vi "流量计UI.vi"() -> ()   [LabVIEW 2016, in "流量计集成.lvlib"]
uses:
  <vilib>/Plasmionique/MB Master/MB_Master_Serial/MB_Master_Serial.lvclass
  C:/Program Files (x86)/National Instruments/LabVIEW 2016/vi.lib/Plasmionique/MB Master/MB_Master/MB_Master.lvclass
  <vilib>/Analysis/baseanly.llb/Mean (DBL).vi
  <vilib>/Utility/config.llb/NI_LVConfig.lvlib
  <vilib>/Analysis/NI_AALBase.lvlib
panel:
  in  "流量计启用 4":bool
  in  "数量 4":u16
  out "流量计类型 4":T1=enum."博意达流量计"
  out "平均水位":dbl
  out "总累积流量":dbl
  out "平均流速":dbl
  out "总流量":dbl
  in  "选项卡控件":T2(tab)
  out "数组":T3[](array[typedef])
  out "数组 2":T4[](array[typedef]) {"累积流量单位" items=["L", "M3", "T", "USG"]; "瞬时流量单位" items=["L/S", "L/M", "L/H", "M3/S", "M3/M", "M3/H", "T/S", "T/M", "T/H", "GPS", "GPM", "GPH"]}
  out "数组 3":T7[](array[typedef])
  out "数组 4":T3[](array[typedef])
  out "MB_Serial session":refnum<class "MB_Master_Serial.lvclass">
  in  "斯坦道功率测流":bool
  in  "流量计启用 3":bool
  in  "数量 3":u16
  out "流量计类型 3":T1=enum."斯坦道功率测流"
  in  "流量计启用 2":bool
  in  "数量 2":u16
  out "流量计类型 2":T1=enum."MGG/KL QC"
  in  "数量":u16
  out "流量计类型":T1
  in  "流量计启用":bool
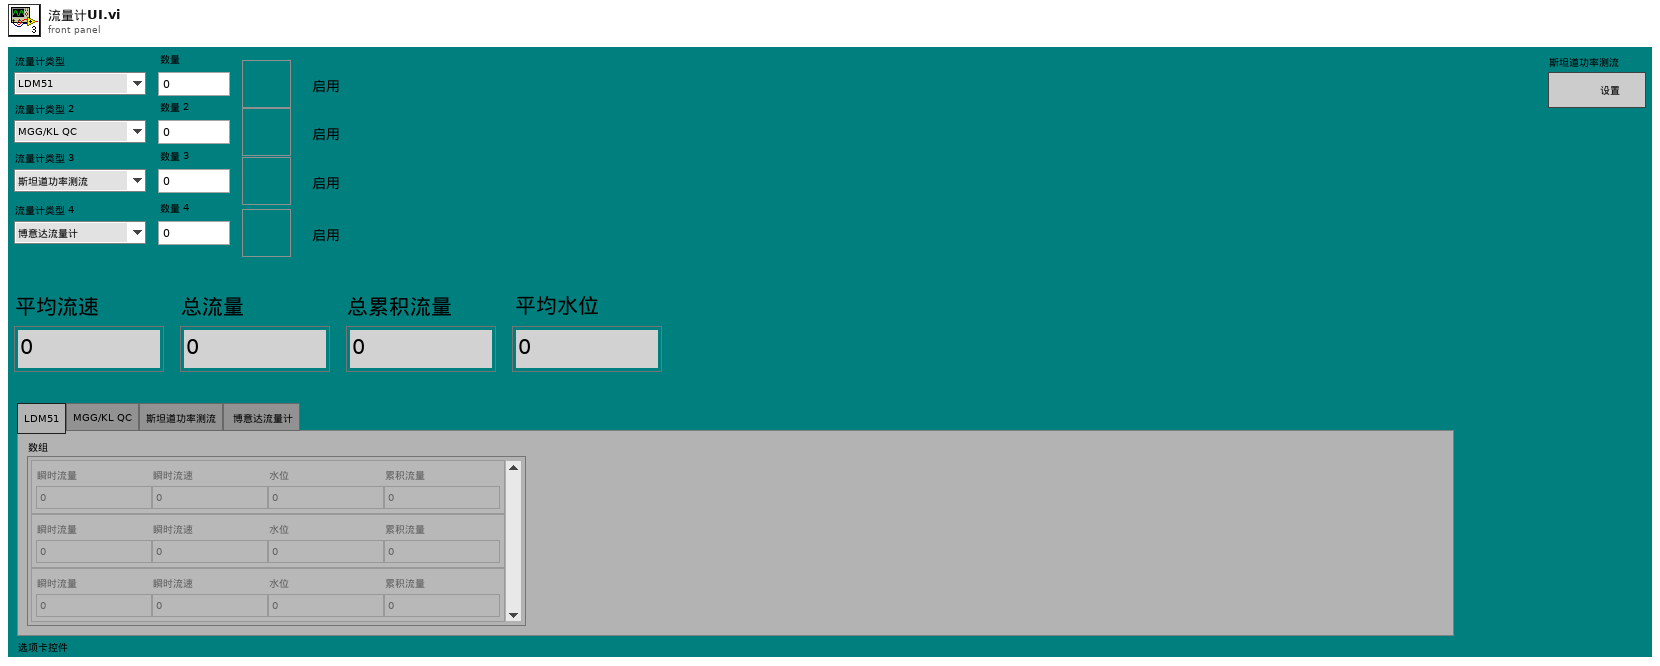
[diagram p1: front panel]
types:
  T1 = typedef "流量计集成.lvlib/流量计类型.ctl" = enum16{"LDM51", "MGG/KL QC", "斯坦道功率测流", "博意达流量计"}
  T2 = enum32{"LDM51", "MGG/KL QC", "斯坦道功率测流", " 博意达流量计"}
  T3 = typedef "流量计集成.lvlib/LDM51明渠流量计.lvlib/读取值.ctl" = cluster{"瞬时流量":sgl, "瞬时流速":sgl, "水位":sgl, "累积流量":sgl}
  T4 = typedef "流量计集成.lvlib/MGG-KL-QC流量计.lvlib/读取值.ctl" = cluster{"瞬时流量":sgl, "瞬时流速":sgl, "流量百分比":sgl, "流体电导比":sgl, "正向累积数值":sgl, "反向累积数值":sgl, "瞬时流量单位":T5, "累积流量单位":T6, "上限报警":u16, "下限报警":u16, "空管报警":u16, "系统报警":u16}
  T5 = typedef "流量计集成.lvlib/MGG-KL-QC流量计.lvlib/瞬时流量单位.ctl" = u16
  T6 = typedef "流量计集成.lvlib/MGG-KL-QC流量计.lvlib/累积流量单位.ctl" = u16
  T7 = typedef "流量计集成.lvlib/斯坦道功率测流.lvlib/状态值.ctl" = cluster{"1号瞬时流量":dbl, "2号瞬时流量":dbl, "3号瞬时流量":dbl, "4号瞬时流量":dbl, "5号瞬时流量":dbl, "6号瞬时流量":dbl, "1号累积流量":dbl, "2号累积流量":dbl, "3号累积流量":dbl, "4号累积流量":dbl, "5号累积流量":dbl, "6号累积流量":dbl, "总瞬时流量":dbl, "总累积流量":dbl}
  T8 = cluster{"时间标识":timestamp, "测量模式":string, "数据类型":string, "监测值":sgl, "单位":string, "数据标识":string, "因子编码":string}
  T9 = typedef "LVDateTimeRec.ctl" = cluster{"秒数的小数部分":dbl, "秒":i32, "分":i32, "时":i32, "日":i32, "月":i32, "年":i32, "天数（周）":i32, "天数（年）":i32, "DST":i32}
  T10 = typedef "流量计集成.lvlib/博意达流量计.lvlib/读取值.ctl" = cluster{"瞬时流量":sgl, "瞬时流速":sgl, "水位":sgl, "累积流量":sgl}
  T11 = typedef "NI_LVConfig.lvlib/Config Data RefNum.ctl" = refnum<k1>
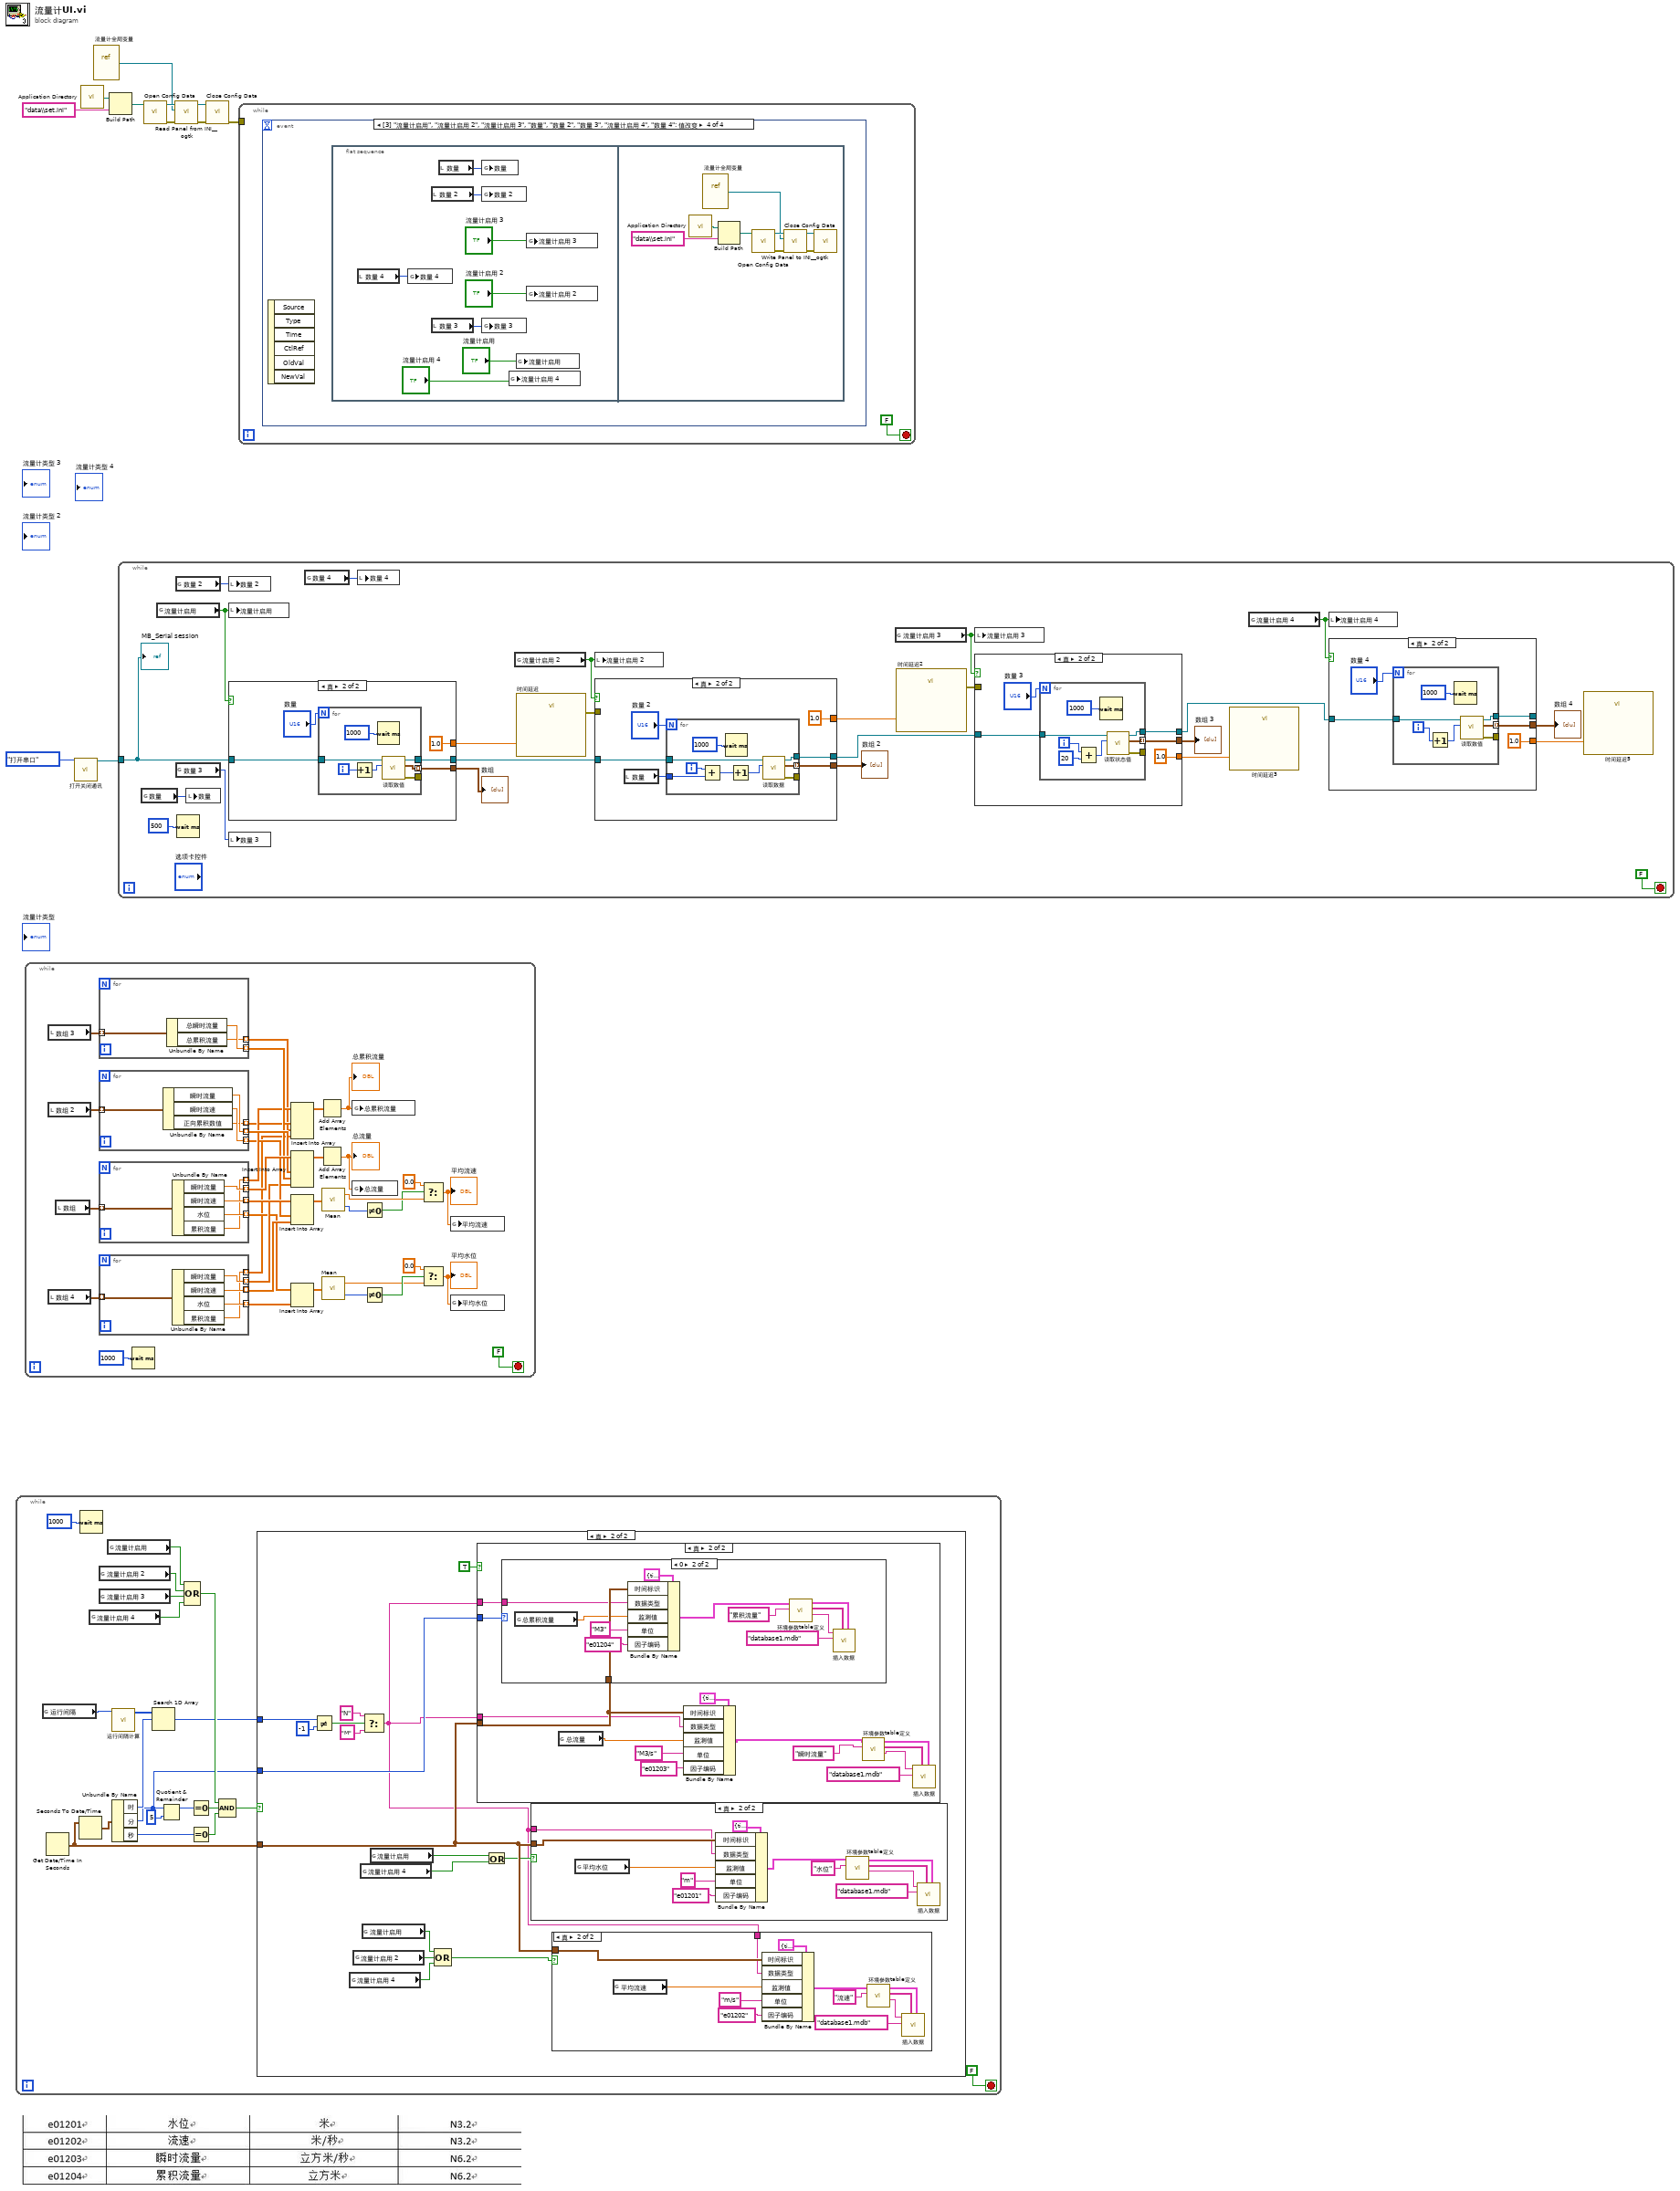
[diagram p0: block diagram]
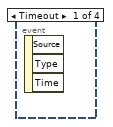
[diagram p7: hidden frame]
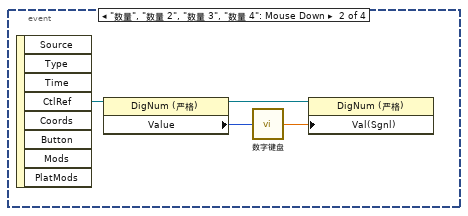
[diagram p8: hidden frame]
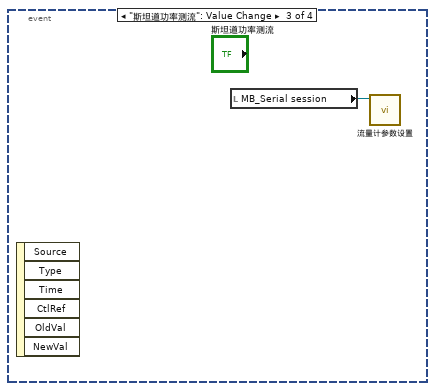
[diagram p9: hidden frame]
diagram:
  n1 = while {
    stop <- FALSE stop-if-true
    n2 = global read "流量计全局变量.vi" "运行间隔"() -> (w13:i16)
    n3 = Get Date/Time In Seconds() -> (seconds since 1Jan1904=w30:timestamp)
    n4 = Seconds To Date/Time(time stamp (now)=w30) -> (date time rec=w29:T9)  [unwired: 1 in]
    n5 = Wait (ms)(milliseconds to wait=u32 1000 ("等待时间（毫秒）")) -> ()  [unwired: 1 out]
    n6 = global read "流量计全局变量.vi" "流量计启用 4"() -> (w12:bool)
    n7 = global read "流量计全局变量.vi" "流量计启用 2"() -> (w20:bool)
    n8 = global read "流量计全局变量.vi" "流量计启用 3"() -> (w19:bool)
    n9 = global read "流量计全局变量.vi" "流量计启用"() -> (w21:bool)
    n10 = call "运行间隔计算.vi"("运行周期"=w13) -> ("数组"=w16:i32[])  [unwired: 10 in]
    n11 = Unbundle By Name(w29) -> ("时"=w17:i32, "分"=w14:i32, "秒"=w27:i32)
    n12 = Search 1D Array(1D array=w16, element=w17) -> (index of element=w15:i32)  [unwired: 1 in]
    n13 = Quotient & Remainder(x=w14, y=5) -> (x-y*floor(x/y)=w26:i32)  [unwired: 1 out]
    n14 = Compound Arithmetic op=OR ("复合运算")(w21, w20, w19, w12) -> (w18:bool)
    n15 = Equal To 0?(x=w26) -> (x = 0?=w25:bool)
    n16 = Equal To 0?(x=w27) -> (x = 0?=w24:bool)
    n17 = Compound Arithmetic op=AND ("复合运算")(w18, w25, w24) -> (w23:bool)
    n18 = case shown="真" w23 {
      tunnel: w30 -> [_ w47]
      tunnel: w15 -> [_ w38]
      tunnel: w14 -> [_ w37]
      frame False {
      }
      frame True {
        n19 = Not Equal?(x=w38, y=-1) -> (x != y?=w41:bool)
        n20 = global read "流量计全局变量.vi" "流量计启用 4"() -> (w35:bool)
        n21 = global read "流量计全局变量.vi" "流量计启用 2"() -> (w43:bool)
        n22 = global read "流量计全局变量.vi" "流量计启用 4"() -> (w33:bool)
        n23 = global read "流量计全局变量.vi" "流量计启用"() -> (w44:bool)
        n24 = Select(t="N" ("单位"), s=w41, f="M" ("单位")) -> (s? t:f=w36:string)
        n25 = global read "流量计全局变量.vi" "流量计启用"() -> (w46:bool)
        n26 = Compound Arithmetic op=OR ("复合运算")(w44, w43, w35) -> (w32:bool)
        n27 = case shown="真" TRUE {
          tunnel: w47 -> [_ w68]
          tunnel: w36 -> [_ w72]
          tunnel: w37 -> [_ w71]
          tunnel: w36 -> [_ w66]
          frame False {
          }
          frame True {
            n28 = case shown="0" w71 {
              tunnel: w68 -> [_ w84]
              tunnel: w72 -> [_ w81]
              frame Default {
              }
              frame 0 {
                n29 = global read "流量计全局变量.vi" "总累积流量"() -> (w82:dbl)
                n30 = Bundle By Name(cluster=T8 {"时间标识"=timestamp(0 s since 1904-01-01), "测量模式"="水样测试", "数据类型"="N", "监测值"=0.0, "单位"="mg/L", "数据标识"="N", "因子编码"=""} ("data"), "时间标识"=w84, "数据类型"=w81, "监测值"=w82, "单位"="M3", "因子编码"="e01204") -> (w78:T8)
                n31 = call "环境参数table定义.vi"("table 输入"="累积流量", "data"=w78) -> ("table 输出"=w74:string, "columns"=w75:string[], "data输出"=w76:T8)  [unwired: 7 in]
                n32 = call "插入数据.vi"("data"=w76, "columns"=w75, "database"="database1.mdb" ("table 输入"), "table"=w74) -> ()  [unwired: 7 in, 1 out]
              }
            }
            n33 = global read "流量计全局变量.vi" "总流量"() -> (w67:dbl)
            n34 = Bundle By Name(cluster=T8 {"时间标识"=timestamp(0 s since 1904-01-01), "测量模式"="水样测试", "数据类型"="N", "监测值"=0.0, "单位"="mg/L", "数据标识"="N", "因子编码"=""} ("data"), "时间标识"=w68, "数据类型"=w66, "监测值"=w67, "单位"="M3/s", "因子编码"="e01203") -> (w64:T8)
            n35 = call "环境参数table定义.vi"("table 输入"="瞬时流量", "data"=w64) -> ("table 输出"=w60:string, "columns"=w61:string[], "data输出"=w62:T8)  [unwired: 7 in]
            n36 = call "插入数据.vi"("data"=w62, "columns"=w61, "database"="database1.mdb" ("table 输入"), "table"=w60) -> ()  [unwired: 7 in, 1 out]
          }
        }
        n37 = Or(x=w46, y=w33) -> (x .or. y?=w45:bool)
        n38 = case shown="真" w45 {
          tunnel: w47 -> [_ w55]
          tunnel: w36 -> [_ w54]
          frame False {
          }
          frame True {
            n39 = global read "流量计全局变量.vi" "平均水位"() -> (w53:dbl)
            n40 = Bundle By Name(cluster=T8 {"时间标识"=timestamp(0 s since 1904-01-01), "测量模式"="水样测试", "数据类型"="N", "监测值"=0.0, "单位"="mg/L", "数据标识"="N", "因子编码"=""} ("data"), "时间标识"=w55, "数据类型"=w54, "监测值"=w53, "单位"="m", "因子编码"="e01201") -> (w49:T8)
            n41 = call "环境参数table定义.vi"("table 输入"="水位", "data"=w49) -> ("table 输出"=w50:string, "columns"=w51:string[], "data输出"=w52:T8)  [unwired: 7 in]
            n42 = call "插入数据.vi"("data"=w52, "columns"=w51, "database"="database1.mdb" ("table 输入"), "table"=w50) -> ()  [unwired: 7 in, 1 out]
          }
        }
        n43 = case shown="真" w32 {
          tunnel: w47 -> [_ w92]
          tunnel: w36 -> [_ w91]
          frame False {
          }
          frame True {
            n44 = global read "流量计全局变量.vi" "平均流速"() -> (w93:dbl)
            n45 = Bundle By Name(cluster=T8 {"时间标识"=timestamp(0 s since 1904-01-01), "测量模式"="水样测试", "数据类型"="N", "监测值"=0.0, "单位"="mg/L", "数据标识"="N", "因子编码"=""} ("data"), "时间标识"=w92, "数据类型"=w91, "监测值"=w93, "单位"="m/s", "因子编码"="e01202") -> (w89:T8)
            n46 = call "环境参数table定义.vi"("table 输入"="流速", "data"=w89) -> ("table 输出"=w86:string, "columns"=w87:string[], "data输出"=w88:T8)  [unwired: 7 in]
            n47 = call "插入数据.vi"("data"=w88, "columns"=w87, "database"="database1.mdb" ("table 输入"), "table"=w86) -> ()  [unwired: 7 in, 1 out]
          }
        }
      }
    }
  }
  n48 = while {
    stop <- FALSE stop-if-true
    n49 = local read "数组 3"() -> (w128:T7[])
    n50 = local read "数组 2"() -> (w129:T4[])
    n51 = local read "数组 4"() -> (w104:T3[])
    n52 = local read "数组"() -> (w132:T3[])
    n53 = for {
      tunnel: w128 -> [w140] mode=indexing
      tunnel: [w139] -> w125 mode=indexing
      tunnel: [w138] -> w122 mode=indexing
      n54 = Unbundle By Name(w140) -> ("总瞬时流量"=w139:dbl, "总累积流量"=w138:dbl)
    }
    n55 = for {
      tunnel: w129 -> [w144] mode=indexing
      tunnel: [w143] -> w126 mode=indexing
      tunnel: [w142] -> w118 mode=indexing
      tunnel: [w141] -> w123 mode=indexing
      n56 = Unbundle By Name(w144) -> ("瞬时流量"=w143:sgl, "瞬时流速"=w142:sgl, "正向累积数值"=w141:sgl)
    }
    n57 = for {
      tunnel: w132 -> [w149] mode=indexing
      tunnel: [w148] -> w127 mode=indexing
      tunnel: [w147] -> w119 mode=indexing
      tunnel: [w146] -> w101 mode=indexing
      tunnel: [w145] -> w124 mode=indexing
      n58 = Unbundle By Name(w149) -> ("瞬时流量"=w148:sgl, "瞬时流速"=w147:sgl, "水位"=w146:sgl, "累积流量"=w145:sgl)
    }
    n59 = for {
      tunnel: w104 -> [w137] mode=indexing
      tunnel: [w136] -> w102 mode=indexing
      tunnel: [w135] -> w103 mode=indexing
      tunnel: [w134] -> w99 mode=indexing
      tunnel: [w133] -> w98 mode=indexing
      n60 = Unbundle By Name(w137) -> ("瞬时流量"=w136:sgl, "瞬时流速"=w135:sgl, "水位"=w134:sgl, "累积流量"=w133:sgl)
    }
    n61 = Wait (ms)(milliseconds to wait=u32 1000 ("等待时间（毫秒）")) -> ()  [unwired: 1 out]
    n62 = Insert Into Array(array=w124, new element #1=w123, new element #2=w122, new element #3=w98) -> (w120:sgl[])  [unwired: 1 in]
    n63 = Insert Into Array(array=w127, new element #1=w126, new element #2=w125, new element #3=w102) -> (w121:sgl[])  [unwired: 1 in]
    n64 = Insert Into Array(array=w119, new element #1=w118, new element #2=w103) -> (w113:sgl[])  [unwired: 1 in]
    n65 = Insert Into Array(array=w101, new element=w99) -> (w100:sgl[])  [unwired: 1 in]
    n66 = Add Array Elements(numeric array=w120) -> (sum=w106:sgl)
    "总累积流量" <- w106
    n67 = Add Array Elements(numeric array=w121) -> (sum=w108:sgl)
    "总流量" <- w108
    n68 = call-poly <vilib>:"Mean.vi"("X"=w113) -> ("mean"=w117:dbl, "error"=w114:i32)
    n69 = call-poly <vilib>:"Mean.vi"("X"=w100) -> ("mean"=w109:dbl, "error"=w112:i32)
    n70 = global write "流量计全局变量.vi" "总累积流量"(w106) -> ()
    n71 = global write "流量计全局变量.vi" "总流量"(w108) -> ()
    n72 = Not Equal To 0?(x=w114) -> (x != 0?=w115:bool)
    n73 = Not Equal To 0?(x=w112) -> (x != 0?=w111:bool)
    n74 = Select(t=0.0, s=w115, f=w117) -> (s? t:f=w107:dbl)
    "平均流速" <- w107
    n75 = Select(t=0.0, s=w111, f=w109) -> (s? t:f=w105:dbl)
    "平均水位" <- w105
    n76 = global write "流量计全局变量.vi" "平均流速"(w107) -> ()
    n77 = global write "流量计全局变量.vi" "平均水位"(w105) -> ()
  }
  n78 = call "打开关闭通讯.vi"("功能输入"=enum16{"打开串口", "关闭串口"}."打开串口") -> ("MB_Serial session"=w1:refnum<class "MB_Master_Serial.lvclass">)  [unwired: 9 in, 1 out]
  n79 = call <vilib>:"Application Directory.vi"() -> ("Application Directory"=w9:path)
  n80 = vi-ref "流量计全局变量.vi"() -> (w3:refnum<vi>)
  n81 = Build Path(base path=w9, name or relative path="data\\set.ini" ("名称或相对路径")) -> (appended path=w10:path)
  n82 = while {
    tunnel: w1 -> [w163]
    stop <- FALSE stop-if-true
    n83 = global read "流量计全局变量.vi" "数量"() -> (w162:u16)
    n84 = global read "流量计全局变量.vi" "流量计启用"() -> (w171:bool)
    n85 = global read "流量计全局变量.vi" "数量 2"() -> (w161:u16)
    n86 = global read "流量计全局变量.vi" "数量 3"() -> (w160:u16)
    n87 = Wait (ms)(milliseconds to wait=u32 500 ("等待时间（毫秒）")) -> ()  [unwired: 1 out]
    n88 = local write "数量"(w162) -> ()
    n89 = local write "数量 2"(w161) -> ()
    n90 = local write "流量计启用"(w171) -> ()
    n91 = case shown="真" w171 {
      tunnel: w163 -> [w217 w222]
      tunnel: [w217 w220] -> w170
      tunnel: [_ w219] -> w168
      tunnel: [_ 1.0 ("Delay Time (s)")] -> w159
      frame False {
      }
      frame True {
        n92 = for {
          N: "数量" -> [_]
          tunnel: w222 -> [w229]
          tunnel: [w228] -> _
          tunnel: [w225] -> w220
          tunnel: [w224] -> w219 mode=indexing
          i -> [w227]
          n93 = Increment(x=w227) -> (x+1=w226:i32)
          n94 = Wait (ms)(milliseconds to wait=u32 1000 ("等待时间（毫秒）")) -> ()  [unwired: 1 out]
          n95 = call "读取数值.vi"("Slave ID"=w226, "MB session in"=w229) -> ("error out"=w228:errorcluster, "读取值"=w224:T3, "MB session out"=w225:refnum<class "MB_Master_Serial.lvclass">)  [unwired: 7 in]
        }
      }
    }
    "数组" <- w168
    n96 = local write "数量 3"(w160) -> ()
    n97 = global read "流量计全局变量.vi" "数量 4"() -> (w150:u16)
    n98 = local write "数量 4"(w150) -> ()
    n99 = global read "流量计全局变量.vi" "流量计启用 2"() -> (w169:bool)
    n100 = call "时间延迟"("Delay Time (s)"=w159) -> ("error out"=w158:errorcluster)  [unwired: 10 in]
    n101 = local write "流量计启用 2"(w169) -> ()
    n102 = case shown="真" w169 {
      tunnel: w170 -> [w201 w206]
      tunnel: [w201 w204] -> w166
      tunnel: [_ w203] -> w167
      tunnel: w158 -> [_ _]
      tunnel: [_ 1.0 ("Delay Time (s)")] -> w157
      frame False {
      }
      frame True {
        n103 = local read "数量"() -> (w205:u16)
        n104 = for {
          N: "数量 2" -> [_]
          tunnel: w206 -> [w215]
          tunnel: w205 -> [w212]
          tunnel: [w211] -> w204
          tunnel: [w210] -> w203 mode=indexing
          tunnel: [w209] -> _
          i -> [w213]
          n105 = Add(x=w213, y=w212) -> (x+y=w214:i32)
          n106 = Wait (ms)(milliseconds to wait=u32 1000 ("等待时间（毫秒）")) -> ()  [unwired: 1 out]
          n107 = Increment(x=w214) -> (x+1=w216:i32)
          n108 = call "读取数据.vi"("Slave ID"=w216, "MB session in"=w215) -> ("error out"=w209:errorcluster, "读取值"=w210:T4, "MB session out"=w211:refnum<class "MB_Master_Serial.lvclass">)  [unwired: 6 in, 1 out]
        }
      }
    }
    "数组 2" <- w167
    n109 = global read "流量计全局变量.vi" "流量计启用 3"() -> (w165:bool)
    n110 = call "时间延迟2"("Delay Time (s)"=w157) -> ("error out"=w155:errorcluster)  [unwired: 10 in]
    n111 = local write "流量计启用 3"(w165) -> ()
    n112 = case shown="真" w165 {
      tunnel: w166 -> [w187 w192]
      tunnel: [w187 w191] -> w152
      tunnel: [_ w189] -> w164
      tunnel: [_ 1.0 ("Delay Time (s)")] -> w156
      tunnel: w155 -> [_ _]
      frame False {
      }
      frame True {
        n113 = for {
          N: "数量 3" -> [_]
          tunnel: w192 -> [w198]
          tunnel: [w195] -> w191
          tunnel: [w196] -> _
          tunnel: [w194] -> w189 mode=indexing
          i -> [w200]
          n114 = Add(x=w200, y=20) -> (x+y=w197:i32)
          n115 = Wait (ms)(milliseconds to wait=u32 1000 ("等待时间（毫秒）")) -> ()  [unwired: 1 out]
          n116 = call "读取状态值.vi"("Slave ID"=w197, "MB session in"=w198) -> ("error out"=w196:errorcluster, "状态值"=w194:T7, "MB session out"=w195:refnum<class "MB_Master_Serial.lvclass">)  [unwired: 6 in, 1 out]
        }
      }
    }
    "数组 3" <- w164
    n117 = call "时间延迟3"("Delay Time (s)"=w156) -> ()  [unwired: 10 in, 1 out]
    n118 = global read "流量计全局变量.vi" "流量计启用 4"() -> (w153:bool)
    n119 = local write "流量计启用 4"(w153) -> ()
    n120 = case shown="真" w153 {
      tunnel: w152 -> [w174 w179]
      tunnel: [w174 w178] -> _
      tunnel: [_ w177] -> w151
      tunnel: [_ 1.0 ("Delay Time (s)")] -> w154
      frame False {
      }
      frame True {
        n121 = for {
          N: "数量 4" -> [_]
          tunnel: w179 -> [w186]
          tunnel: [w184] -> w178
          tunnel: [w185] -> _
          tunnel: [w183] -> w177 mode=indexing
          i -> [w181]
          n122 = Increment(x=w181) -> (x+1=w180:i32)
          n123 = Wait (ms)(milliseconds to wait=u32 1000 ("等待时间（毫秒）")) -> ()  [unwired: 1 out]
          n124 = call "读取数值.vi"("Slave ID"=w180, "MB session in"=w186) -> ("error out"=w185:errorcluster, "读取值"=w183:T10, "MB session out"=w184:refnum<class "MB_Master_Serial.lvclass">)  [unwired: 7 in]
        }
      }
    }
    "数组 4" <- w151
    n125 = call "时间延迟5"("Delay Time (s)"=w154) -> ()  [unwired: 10 in, 1 out]
    "MB_Serial session" <- w163
  }
  n126 = call <vilib>:"Open Config Data.vi"("configuration file path"=w10) -> ("error out"=w7:errorcluster, "refnum"=w8:T11)  [unwired: 8 in, 1 out]
  n127 = call <userlib>:"Read Panel from INI__ogtk.vi"("error in (no error)"=w7, "VI ref"=w3, "refnum"=w8) -> ("error out"=w5:errorcluster, "refnum out"=w6:T11)  [unwired: 7 in]
  n128 = call <vilib>:"Close Config Data.vi"("error in (no error)"=w5, "refnum"=w6) -> ("error out"=w4:errorcluster)  [unwired: 8 in, 1 out]
  n129 = while {
    tunnel: w4 -> [_]
    stop <- FALSE stop-if-true
    n130 = event shown="[3] \"流量计启用\", \"流量计启用 2\", \"流量计启用 3\", \"数量\", \"数量 2\", \"数量 3\", \"流量计启用 4\", \"数量 4\": 值改变" {
      selector: _ -> [_ _ _ _]
      dyn-events: _ -> [_ _ _ _]
      timeout: _ -> [_ _ _ _]
      event Timeout {
        n131 = event-data() -> ()  [unwired: 1 in, 3 out]
      }
      event "数量", "数量 2", "数量 3", "数量 4": Mouse Down {
        n132 = event-data() -> ("CtlRef"=w234:refnum<vi>)  [unwired: 1 in, 7 out]
        n133 = property class="DigNum (严格)"(reference=w234) -> (reference out=w232:refnum<vi>, "Value"=w233:u16)  [unwired: 1 in, 1 out]
        n134 = call "数字键盘.vi"("OldNumber"=w233) -> ("NewNumber"=w231:dbl)
        n135 = property class="DigNum (严格)"(reference=w232, "Val(Sgnl)"=w231) -> ()  [unwired: 1 in, 2 out]
      }
      event "斯坦道功率测流": Value Change {
        n136 = event-data() -> ()  [unwired: 1 in, 6 out]
        n137 = local read "MB_Serial session"() -> (w235:refnum<class "MB_Master_Serial.lvclass">)
        n138 = call "流量计参数设置.vi"("MB session in"=w235) -> ()  [unwired: 11 in]
      }
      event "流量计启用", "流量计启用 2", "流量计启用 3", "数量", "数量 2", "数量 3", "流量计启用 4", "数量 4": Value Change {
        n139 = event-data() -> ()  [unwired: 1 in, 6 out]
        n140 = flat-sequence {
          frame #0 {
            n141 = local read "数量 4"() -> (w236:u16)
            n142 = global write "流量计全局变量.vi" "数量 4"(w236) -> ()
            n143 = local read "数量 2"() -> (w239:u16)
            n144 = local read "数量 3"() -> (w238:u16)
            n145 = local read "数量"() -> (w240:u16)
            n146 = global write "流量计全局变量.vi" "数量"(w240) -> ()
            n147 = global write "流量计全局变量.vi" "数量 2"(w239) -> ()
            n148 = global write "流量计全局变量.vi" "数量 3"(w238) -> ()
            n149 = global write "流量计全局变量.vi" "流量计启用 4"("流量计启用 4") -> ()
            n150 = global write "流量计全局变量.vi" "流量计启用"("流量计启用") -> ()
            n151 = global write "流量计全局变量.vi" "流量计启用 3"("流量计启用 3") -> ()
            n152 = global write "流量计全局变量.vi" "流量计启用 2"("流量计启用 2") -> ()
          }
          frame #1 {
            n153 = call <vilib>:"Application Directory.vi"() -> ("Application Directory"=w247:path)
            n154 = vi-ref "流量计全局变量.vi"() -> (w244:refnum<vi>)
            n155 = Build Path(base path=w247, name or relative path="data\\set.ini" ("名称或相对路径")) -> (appended path=w246:path)
            n156 = call <vilib>:"Open Config Data.vi"("configuration file path"=w246) -> ("error out"=w249:errorcluster, "refnum"=w251:T11)  [unwired: 8 in, 1 out]
            n157 = call <userlib>:"Write Panel to INI__ogtk.vi"("error in (no error)"=w249, "VI ref"=w244, "refnum"=w251) -> ("error out"=w248:errorcluster, "refnum out"=w250:T11)  [unwired: 7 in]
            n158 = call <vilib>:"Close Config Data.vi"("error in (no error)"=w248, "refnum"=w250) -> ()  [unwired: 8 in, 2 out]
          }
        }
      }
    }
  }
